vi "write_tiff.vi"() -> ()   [LabVIEW 2013]
uses:
  <vilib>/vision/NI_Vision_Development_Module.lvlib
panel:
  out "size(s)":i32[](array[numeric])
  out "frame_data_offset":u32
  out "appended path":path
  out "next_IFD_offset_offset":u32
  in  "description":string
  in  "image_length":u32
  in  "image_width":u32
  out "temp_tiff_file":refnum<file>
  out "byteorder":T1(ring)=enum."little-endian"
  in  "filetype":enum16{"motorola", "intel"}(ring)
  in  "Tab Control":enum32{"Page 1", "Page 2"}(tab)
  out "Image":T2(plugin-control)
  out "type3_U16":u16
  out "type4_U32":u32
  in  "byte order":T1(ring)
  out "tif_file":refnum<file>
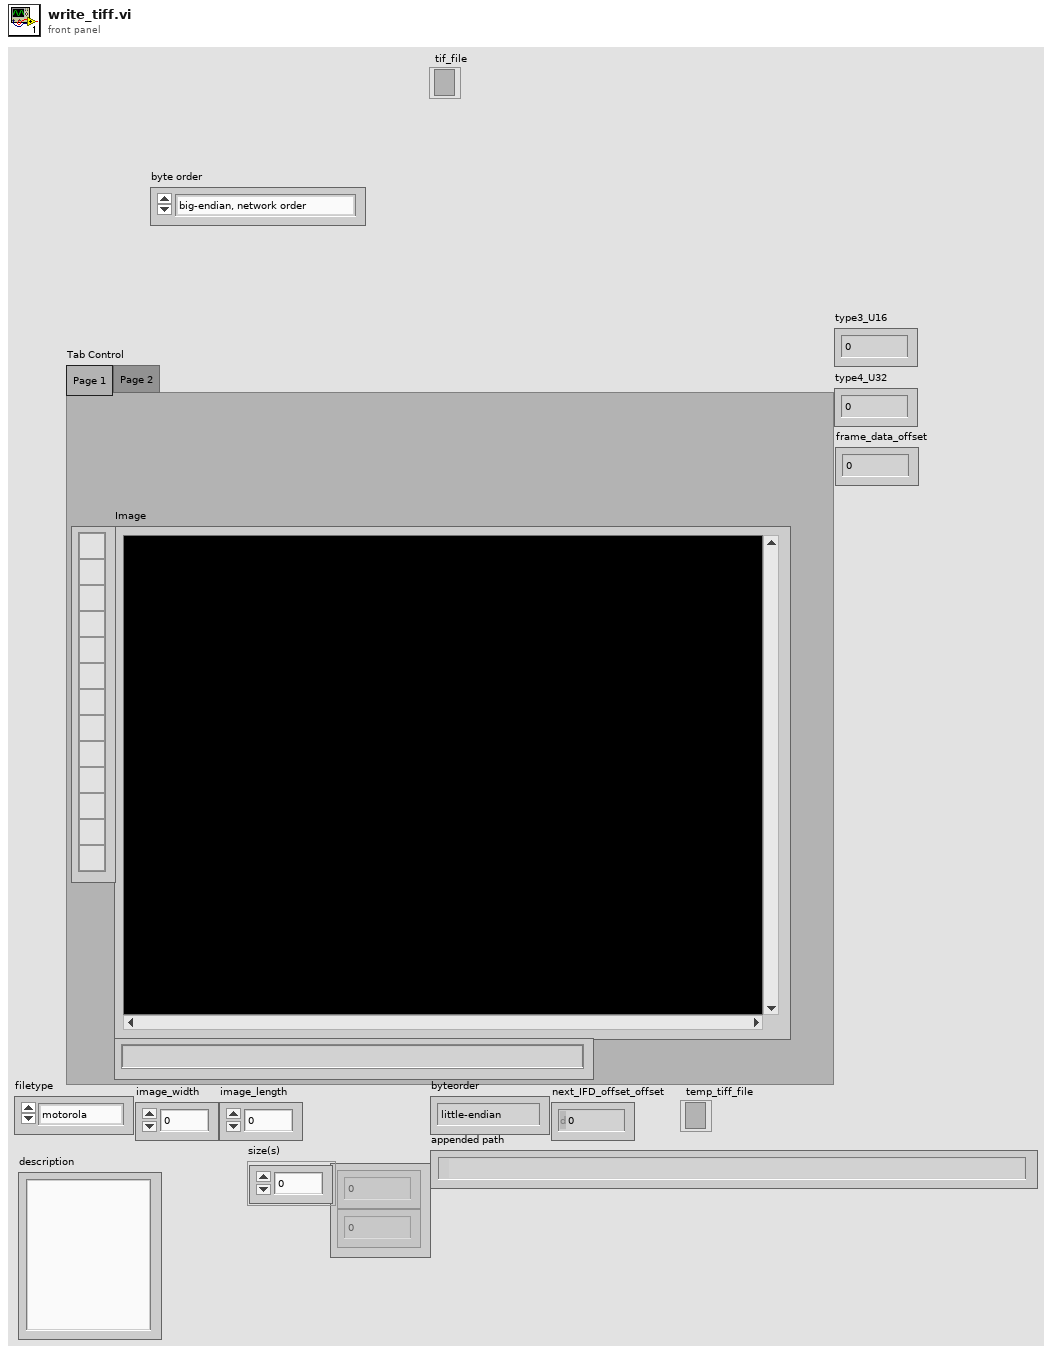
[diagram p1: front panel]
types:
  T1 = enum16{"big-endian, network order", "native, host order", "little-endian"}
  T2 = typedef "IMAQ Image.ctl" = refnum<image>
  T3 = enum16{"open", "replace", "create", "open or create", "replace or create", "replace or create with confirmation"}
  T4 = cluster{"BitDeepth":enum16{"8bit", "16bit", "32bit"}, "image_width":u32, "image_length":u32, "IFD_offset":u32, "description":string}
  T5 = typedef "Image Type" = u32
  T6 = cluster{"byteorder":u16, "version":u16, "Offset_first_IFD":u32}
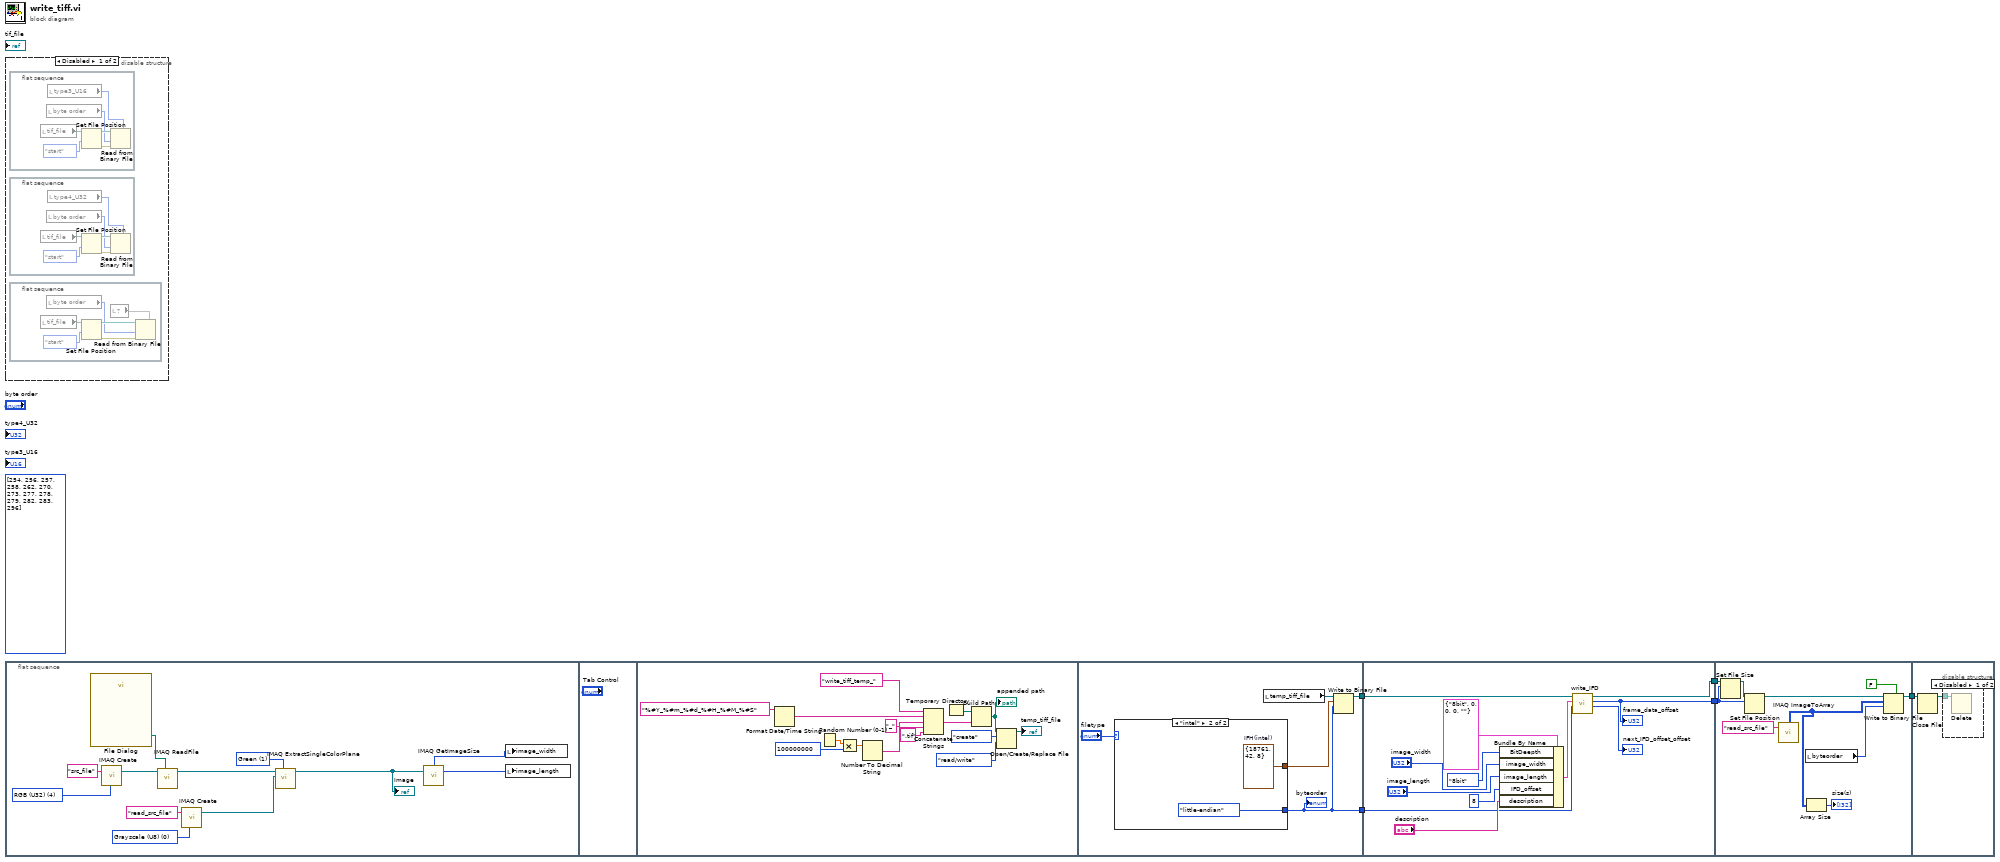
[diagram p0: block diagram]
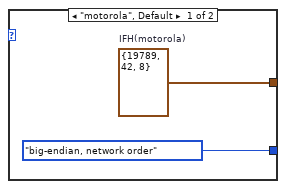
[diagram p2: hidden frame]
diagram:
  (unwired) u16[] [254, 256, 257, 258, 262, 270, 273, 277, 278, 279, 282, 283, 296] ("DE_tag_IDs")
  n1 = disable-structure shown="Disabled" {
    frame Disabled {
      n2 = flat-sequence {
        frame #0 {
          n3 = local read "tif_file"() -> (w17:refnum<file>)
          n4 = local read "byte order"() -> (w13:T1)
          n5 = local read "type3_U16"() -> (w12:u16)
          n6 = Set File Position(refnum=w17, from (0:start)=enum16{"start", "end", "current"}."start") -> (refnum out=w14:refnum<file>, error out=w15:errorcluster)  [unwired: 2 in]
          n7 = Read from Binary File(5:w12, 8:w15, 9:w13, 11:w14) -> ()  [unwired: 2 in, 4 out]
        }
      }
      n8 = flat-sequence {
        frame #0 {
          n9 = local read "tif_file"() -> (w11:refnum<file>)
          n10 = local read "byte order"() -> (w7:T1)
          n11 = local read "type4_U32"() -> (w6:u32)
          n12 = Set File Position(refnum=w11, from (0:start)=enum16{"start", "end", "current"}."start") -> (refnum out=w8:refnum<file>, error out=w9:errorcluster)  [unwired: 2 in]
          n13 = Read from Binary File(5:w6, 8:w9, 9:w7, 11:w8) -> ()  [unwired: 2 in, 4 out]
        }
      }
      n14 = flat-sequence {
        frame #0 {
          n15 = local read "tif_file"() -> (w23:refnum<file>)
          n16 = local read "byte order"() -> (w19:T1)
          n17 = Set File Position(refnum=w23, from (0:start)=enum16{"start", "end", "current"}."start") -> (refnum out=w20:refnum<file>, error out=w21:errorcluster)  [unwired: 2 in]
          n18 = local read item#-1() -> (w18)
          n19 = Read from Binary File(5:w18, 8:w21, 9:w19, 11:w20) -> ()  [unwired: 2 in, 4 out]
        }
      }
    }
    frame Enabled {
    }
  }
  n20 = flat-sequence {
    tunnel: [w51] -> w5
    tunnel: [w52] -> w4
    tunnel: w5 -> [w64]
    tunnel: w4 -> [w63]
    tunnel: [w62] -> w3
    tunnel: [w60] -> w1
    tunnel: w3 -> [w76]
    tunnel: [w79] -> w2
    tunnel: w1 -> [w74]
    tunnel: w2 -> [w82]
    frame #0 {
      w26 = T5 0 items=["Grayscale (U8)", "Grayscale (I16)", "Grayscale (SGL)", "Complex (CSG)", "RGB (U32)", "HSL (U32)", "RGB (U64)", "Grayscale (U16)"] ("Image Type")
      w34 = 1 items=["Red", "Green", "Blue", "Hue", "Saturation", "Luminance", "Value", "Intensity"] ("Color Plane")
      w33 = T5 4 items=["Grayscale (U8)", "Grayscale (I16)", "Grayscale (SGL)", "Complex (CSG)", "RGB (U32)", "HSL (U32)", "RGB (U64)", "Grayscale (U16)"] ("Image Type")
      n21 = call "File Dialog"() -> ("selected path"=w35:path)  [unwired: 12 in, 3 out]
      n22 = call "IMAQ Create"("Image Name"="src_file", "Image Type"=w33) -> ("New Image"=w31:T2)  [unwired: 3 in, 1 out]
      n23 = call "IMAQ ReadFile"("File Path"=w35, "Image"=w31) -> ("Image Out"=w28:T2)  [unwired: 5 in, 4 out]
      n24 = call "IMAQ Create"("Image Name"="read_src_file", "Image Type"=w26) -> ("New Image"=w25:T2)  [unwired: 3 in, 1 out]
      n25 = call "IMAQ ExtractSingleColorPlane"("Color Plane"=w34, "Image Dst"=w25, "Image Src"=w28) -> ("Image Dst Out"=w24:T2)  [unwired: 7 in, 1 out]
      "Image" <- w24
      n26 = call "IMAQ GetImageSize"("Image"=w24) -> ("Y Resolution"=w30:i32, "X Resolution"=w29:i32)  [unwired: 3 in, 1 out]
      n27 = local write "image_width"(w29) -> ()
      n28 = local write "image_length"(w30) -> ()
    }
    frame #1 {
    }
    frame #2 {
      n29 = Format Date/Time String(time format string (%c)="%#Y_%#m_%#d_%#H_%#M_%#S") -> (date/time string=w45:string)  [unwired: 2 in]
      n30 = Random Number (0-1)() -> (number: 0 to 1=w40:dbl)
      n31 = Multiply(x=w40, y=100000000) -> (x*y=w38:dbl)
      n32 = Number To Decimal String(number=w38) -> (decimal integer string=w37:string)  [unwired: 1 in]
      n33 = Concatenate Strings("write_tiff_temp_", w45, "_" ("string"), w37, ".tif" ("string")) -> (w43:string)
      n34 = Temporary Directory() -> (w48:path)
      n35 = Build Path(base path=w48, name or relative path=w43) -> (appended path=w42:path)
      "appended path" <- w42
      n36 = Open/Create/Replace File(file path (use dialog)=w42, operation (0:open)=T3."create", access (0:read/write)=enum16{"read/write", "read-only", "write-only"}."read/write") -> (refnum out=→"temp_tiff_file":refnum<file>)  [unwired: 3 in, 2 out]
    }
    frame #3 {
      n37 = case shown="\"intel\"" "filetype" {
        tunnel: [w57 w59] -> w55
        tunnel: [T1."big-endian, network order" ("byte order (0:big-endian, network order)") T1."little-endian" ("byte order (0:big-endian, network order)")] -> w52
        frame "motorola", Default {
          w57 = T6 {"byteorder"=19789, "version"=42, "Offset_first_IFD"=8}  # IFH(motorola)
        }
        frame "intel" {
          w59 = T6 {"byteorder"=18761, "version"=42, "Offset_first_IFD"=8}  # IFH(intel)
        }
      }
      "byteorder" <- w52
      n38 = local read "temp_tiff_file"() -> (w53:refnum<file>)
      n39 = Write to Binary File(file (use dialog)=w53, data=w55, 9:w52) -> (refnum out=w51:refnum<file>)  [unwired: 3 in, 2 out]
    }
    frame #4 {
      n40 = Bundle By Name(cluster=T4 {"BitDeepth"=enum."8bit", "image_width"=0, "image_length"=0, "IFD_offset"=0, "description"=""} ("Cluster"), "BitDeepth"=enum16{"8bit", "16bit", "32bit"}."8bit", "image_width"="image_width", "image_length"="image_length", "IFD_offset"=u32 8, "description"="description") -> (w65:T4)
      n41 = call "write_IFD.vi"("byte order (0:big-endian, network order)"=w63, "Cluster"=w65, "tiff_file_input"=w64) -> ("next_IFD_offset_offset"=→"next_IFD_offset_offset":u32, "frame_data_offset"=w60:u32, "tiff_file_out"=w62:refnum<file>)  [unwired: 5 in, 1 out]
      "frame_data_offset" <- w60
    }
    frame #5 {
      n42 = Set File Size(6:w74, 7:w76) -> (3:w75:refnum<file>)  [unwired: 1 in, 1 out]
      n43 = Set File Position(offset (in bytes) (0)=w74, refnum=w75) -> (refnum out=w77:refnum<file>)  [unwired: 2 in, 1 out]
      n44 = call "IMAQ ImageToArray"("Image"="read_src_file" ("Image Name")) -> ("Image Pixels (U8)"=w73:u8[][])  [unwired: 3 in, 4 out]
      n45 = local read "byteorder"() -> (w78:T1)
      n46 = Array Size(array=w73) -> (size(s)=→"size(s)":i32[])
      n47 = Write to Binary File(file (use dialog)=w77, data=w73, 5:FALSE ("prepend array or string size? (T)"), 9:w78) -> (refnum out=w79:refnum<file>)  [unwired: 2 in, 2 out]
    }
    frame #6 {
      n48 = Close File(refnum=w82) -> (path=w83:path)  [unwired: 1 in, 1 out]
      n49 = disable-structure shown="Disabled" {
        disable-tunnel: w83 -> [w84 _]
        frame Disabled {
          n50 = Delete(path (use dialog)=w84) -> ()  [unwired: 4 in, 3 out]
        }
        frame Enabled {
        }
      }
    }
  }
